vi "LinxUartRead.vi"(8 "Error In":errorcluster, 9 "Num Bytes":u8, 10 "Uart Channel":u8, 11 "LINX Resource":T1) -> (0 "Error Out":errorcluster, 1 "Num Bytes Read":u8, 2 "Data":u8[](array[numeric]), 3 "LINX Resource":T1)   [LabVIEW 2019, in "LMH-LINX.lvlib" / "Local IO.lvlib"]
uses:
  <vilib>/MakerHub/LINX/Private/Local IO/Local IO.lvlib
  <vilib>/MakerHub/LINX/Private/Type Defs/LINX Ref.ctl
  <vilib>/MakerHub/LINX/Private/Type Defs/Platform.ctl
  <vilib>/MakerHub/LINX/Private/Type Defs/Interface.ctl
  <vilib>/MakerHub/LINX/Private/Device/Type Defs/LINX Device Config.ctl
  <vilib>/MakerHub/LINX/Private/Device/Type Defs/TCP Config.ctl
  <vilib>/MakerHub/LINX/Private/Device/Type Defs/Channels.ctl
  <vilib>/MakerHub/LINX/Private/Type Defs/Error Type.ctl
  <vilib>/MakerHub/LINX/LMH-LINX.lvlib
  <vilib>/MakerHub/LINX/Private/Type Defs/Channel FGV States.ctl
  liblinxdevice.dll
  <vilib>/MakerHub/LINX/Private/Device/Device.lvlib
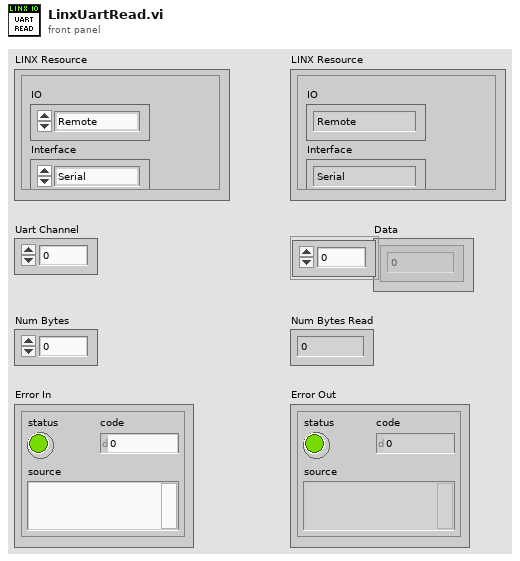
[diagram p1: front panel]
types:
  T1 = typedef "LMH-LINX.lvlib/LINX Ref.ctl" = cluster{"IO":T2, "Interface":T3, "LINX Device Config":T4}
  T2 = typedef "LMH-LINX.lvlib/Platform.ctl" = enum16{"Remote", "Local"}
  T3 = typedef "LMH-LINX.lvlib/Interface.ctl" = enum16{"Serial", "TCP"}
  T4 = typedef "LMH-LINX.lvlib/Device.lvlib/LINX Device Config.ctl" = cluster{"Interface":T3, "COM Port":refnum<visa-resource-name>, "TCP Configuration":T5, "Device Family":u8, "Device ID":u8, "Device Name":string, "TCP Ref":refnum<k5>, "Channels":T6}
  T5 = typedef "LMH-LINX.lvlib/Device.lvlib/TCP Config.ctl" = cluster{"IP Address":string, "Port":u16}
  T6 = typedef "LMH-LINX.lvlib/Channels.ctl" = cluster{"DI":u8[], "DO":u8[], "AI":u8[], "AO":u8[], "PWM":u8[], "QE":u8[], "UART":u8[], "I2C 2":u8[], "SPI":u8[], "CAN":u8[], "Servo":u8[], "AI Ref (V)":dbl, "AI Resolution (Bits)":u8, "AO Ref (V)":dbl, "AO Resolution (Bits)":u8}
  T7 = typedef "LMH-LINX.lvlib/Error Type.ctl" = enum16{"Unknown", "Timeout", "Corrupt Return Packet", "Unable To Connect", "Command Not Supported", "Channel DNE", "Invalid COM Config", "Firmware Version Mismatch", "myRIO Support", "CMD Specific Error", "Local IO Not Supported"}
  T8 = typedef "LMH-LINX.lvlib/Channel FGV States.ctl" = enum16{"Initialize", "Get", "Set"}
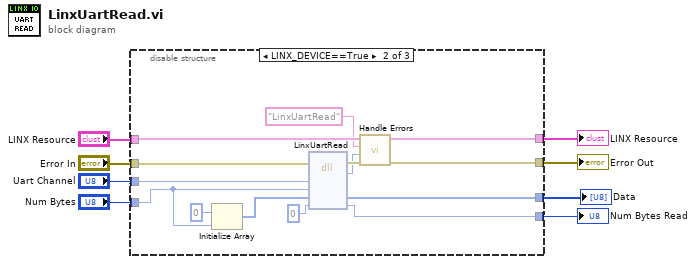
[diagram p0: block diagram]
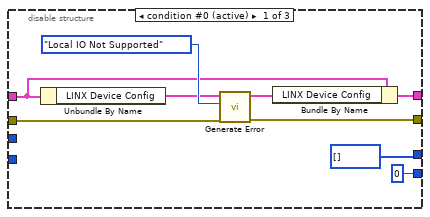
[diagram p2: hidden frame]
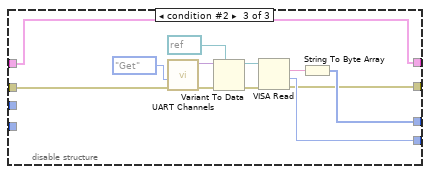
[diagram p3: hidden frame]
diagram:
  n1 = disable-structure shown="LINX_DEVICE==True" {
    disable-tunnel: [w11 w28 w35] -> w7
    disable-tunnel: "LINX Resource" -> [w13 w29 w35]
    disable-tunnel: "Error In" -> [w16 w31 w36]
    disable-tunnel: [w15 w26 w32] -> w8
    disable-tunnel: "Uart Channel" -> [_ w30 _]
    disable-tunnel: "Num Bytes" -> [_ w23 _]
    disable-tunnel: [u8 0 ("Baud Rate") w19 w33] -> w2
    disable-tunnel: [u8[] [] ("Data") w18 w34] -> w1
    frame condition #0 (active) {
      n2 = Unbundle By Name(w13) -> ("LINX Device Config"=w14:T4)
      n3 = call <vilib>:"Generate Error.vi"("Error In"=w16, "Error Type"=Error_Type."Local IO Not Supported", "LINX Device Config"=w14) -> ("Error Out"=w15:errorcluster, "Dup LINX Device Config"=w12:T4)  [unwired: 7 in]
      n4 = Bundle By Name(cluster=w13, "LINX Device Config"=w12) -> (w11:T1)
    }
    frame condition #1 {
      n5 = Initialize Array(u8 0 ("element"), w23) -> (w21:u8[])
      n6 = dll-call lib="liblinxdevice.*" fn="LinxUartRead"(error in=w31, "channel"=w30, "numBytes"=w23, "recBuffer"=w21, "numBytesRead"=u8 0) -> (error out=w27:errorcluster, "status"=w24:i32, "recBuffer"=w18:u8[], "numBytesRead"=w19:u8)  [unwired: 4 in, 1 out]
      n7 = call <vilib>:"Handle Errors.vi"("Error In"=w27, "LinxStatus"=w24, "Function Name"="LinxUartRead", "LINX Resource"=w29) -> ("Error Out"=w26:errorcluster, "LINX Resource"=w28:T1)  [unwired: 6 in]
    }
    frame condition #2 {
      n8 = call <vilib>:"UART Channels.vi"("Error In"=w36, "Channel State"=Channel_FGV_States."Get") -> ("Error Out"=w37:errorcluster, "UART Channel"=w38:variant)  [unwired: 8 in]
      n9 = Variant To Data(error in=w37, type=refnum<visa-resource-name> refnum ("reference"), Variant=w38) -> (data=w41:refnum<visa-resource-name>, error out=w42:errorcluster)
      n10 = VISA Read(VISA resource name=w41, error in (no error)=w42) -> (read buffer=w43:string, return count=w33:u32, error out=w32:errorcluster)  [unwired: 1 in, 1 out]
      n11 = String To Byte Array(string=w43) -> (unsigned byte array=w34:u8[])
    }
  }
  "LINX Resource" <- w7
  "Num Bytes Read" <- w2
  "Error Out" <- w8
  "Data" <- w1
